vi "8021AS Status.vi"(8 "error in (no error)":errorcluster, 11 "Time Reference ID":string="IEEE 802.1AS-2011_1") -> (0 "error out":errorcluster, 1 "Grandmaster ID":string, 2 "State":T1(ring), 3 "Offset (ns)":i64, 4 "Grandmaster MAC address":string, 5 "Time Reference Selected":bool)   [LabVIEW 2017]
doc: "Returns current 802.11AS status visible to a target.\n\nphaseOffset - Offset from the 802.1AS master in nanoseconds.\nstate - PTP state that this target is in.\nGrandmaster ID - Identifier for the 802.1AS grand master.\nGrandmaster MAC sddress - MAC address for the 802.1AS grand master."
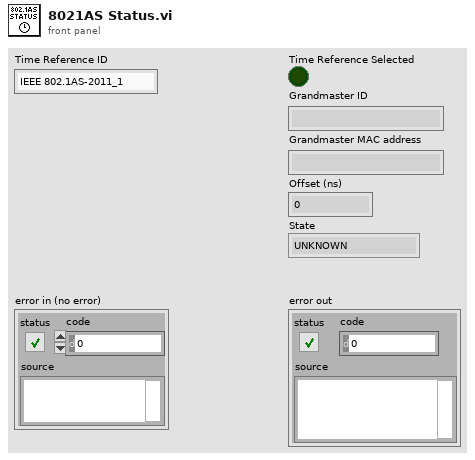
[diagram p1: front panel]
types:
  T1 = enum16{"UNKNOWN", "MASTER", "SLAVE", "DISABLED", "PASSIVE"}
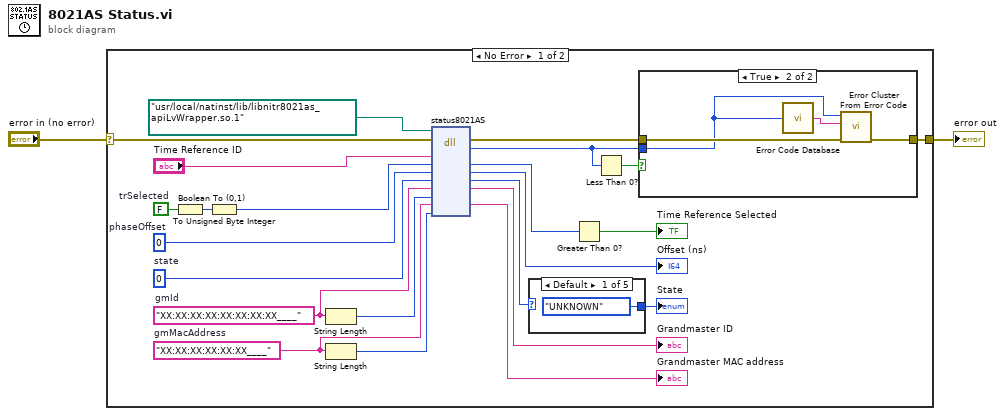
[diagram p0: block diagram]
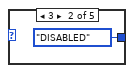
[diagram p2: hidden frame]
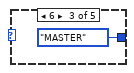
[diagram p3: hidden frame]
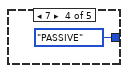
[diagram p4: hidden frame]
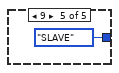
[diagram p5: hidden frame]
diagram:
  n1 = case shown="No Error" "error in (no error)" {
    selector: "error in (no error)" -> [w19 w36]
    tunnel: [w21 w36] -> w1
    frame No Error {
      w7 = FALSE  # trSelected
      w14 = "XX:XX:XX:XX:XX:XX____"  # gmMacAddress
      w16 = "XX:XX:XX:XX:XX:XX:XX:XX____"  # gmId
      w17 = u8 0  # state
      w24 = i64 0  # phaseOffset
      n2 = Boolean To (0,1)(Boolean=w7) -> (0, 1=w6:i16)
      n3 = To Unsigned Byte Integer(number=w6) -> (unsigned 8bit integer=w5:u8)
      n4 = String Length(string=w16) -> (length=w15:i32)
      n5 = String Length(string=w14) -> (length=w13:i32)
      n6 = dll-call lib="usr/local/natinst/lib/libcriochro.so" fn="status8021AS"(path in=path "/usr/local/natinst/lib/libnitr8021as_apiLvWrapper.so.1", error in=w19, "trId"="Time Reference ID", "trSelected"=w5, "phaseOffset"=w24, "state"=w17, "gmId"=w16, "gmIdSize"=w15, "gmMacAddress"=w14, "gmMacAddressSize"=w13) -> (error out=w22:errorcluster, "return type"=w20:i32, "trSelected"=w4:u8, "phaseOffset"=→"Offset (ns)":i64, "state"=w10:u8, "gmId"=→"Grandmaster ID":string, "gmMacAddress"=→"Grandmaster MAC address":string)  [unwired: 4 in, 1 out]
      n7 = case shown="Default" w10 {
        tunnel: [T1."UNKNOWN" ("State") T1."DISABLED" ("State") T1."MASTER" ("State") T1."PASSIVE" ("State") T1."SLAVE" ("State")] -> w9
        frame Default {
        }
        frame 3 {
        }
        frame 6 {
        }
        frame 7 {
        }
        frame 9 {
        }
      }
      "State" <- w9
      n8 = Greater Than 0?(x=w4) -> (x > 0?=→"Time Reference Selected":bool)
      n9 = Less Than 0?(x=w20) -> (x < 0?=w23:bool)
      n10 = case shown="True" w23 {
        tunnel: w22 -> [w31 w35]
        tunnel: [w31 w34] -> w21
        tunnel: w20 -> [_ w32]
        frame False {
        }
        frame True {
          n11 = call <vilib>:"Error Code Database.vi"("Error Code"=w32) -> ("Error Text"=w33:string)
          n12 = call <vilib>:"Error Cluster From Error Code.vi"("error in (no error)"=w35, "error message (\"\")"=w33, "error code (0)"=w32) -> ("error out"=w34:errorcluster)  [unwired: 6 in]
        }
      }
    }
    frame Error {
    }
  }
  "error out" <- w1
